vi "Draw Robot Active Curve.vi"(9 "theta":dbl, 10 "Curvature":dbl, 11 "Cluster":cluster{"x":dbl, "y":dbl}) -> (3 "circle":cluster{dbl[], dbl[]})   [LabVIEW 2017, in "Pure Pursuit.lvlib"]
uses:
  Pure Pursuit.lvlib
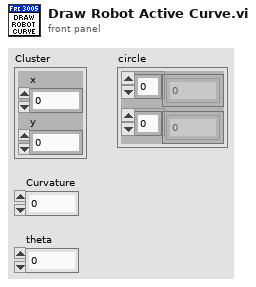
[diagram p1: front panel]
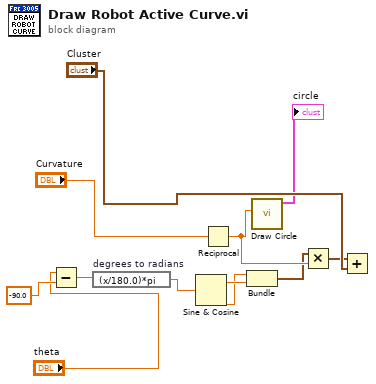
[diagram p0: block diagram]
diagram:
  n1 = Subtract(x="theta", y=-90.0) -> (x-y=w6:dbl)
  n2 = expression code="(x/180.0)*pi" "degrees to radians"(w6) -> (w5:dbl)
  n3 = Sine & Cosine(0:w5) -> (1:w4:dbl, 2:w3:dbl)
  n4 = Reciprocal(x="Curvature") -> (1/x=w11:dbl)
  n5 = Bundle(w3, w4) -> (w10:cluster{dbl, dbl})  [unwired: 1 in]
  n6 = call "Draw Circle.vi"("r"=w11) -> ("circle"=→"circle":cluster{dbl[], dbl[]})  [unwired: 10 in]
  n7 = Multiply(x=w10, y=w11) -> (x*y=w9:cluster{dbl, dbl})
  n8 = Add(x=w9, y="Cluster") -> ()  [unwired: 1 out]
